vi "Initialize.vi"(4 "stop bits (1.0)":u16(ring)=10 items=["1.0"=10, "2.0"=20], 5 "timeout, ms (300)":u32=300, 6 "parity (none)":enum16{"None", "Odd", "Even"}(ring), 7 "address (1)":u8=1, 8 "error in (no error)":errorcluster, 9 "data bits (8)":u16(ring)=8 items=["7"=7, "8"=8], 10 "baud rate (1200)":u32(ring)=1200 items=["600"=600, "1200"=1200, "2400"=2400, "4800"=4800, "9600"=9600, "19200"=19200], 11 "port":refnum<visa-resource-name>) -> (0 "error out":errorcluster, 3 "HECR out":refnum<class "PL SMC HECR.lvclass">)   [LabVIEW 2015, in "PL SMC HECR.lvclass"]
doc: "Initializes connection to device using specified settings."
uses:
  PL SMC HECR.lvclass
  <vilib>/plasmapper/PL Modbus Client/PL Modbus Client.lvclass
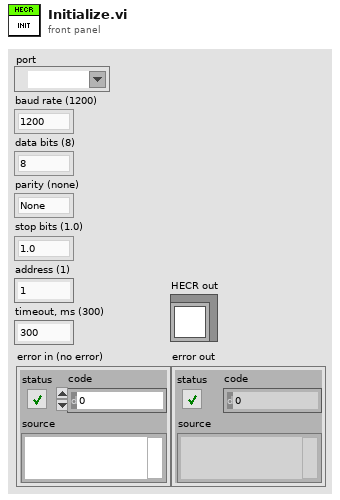
[diagram p1: front panel]
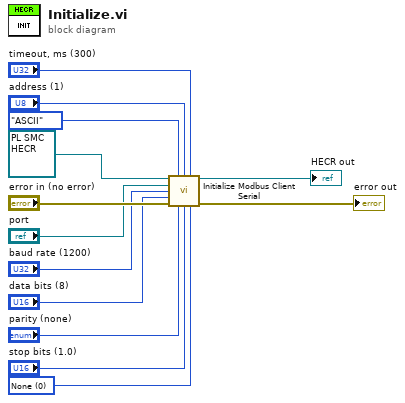
[diagram p0: block diagram]
diagram:
  w9 = u16 0 items=["None", "XON/XOFF", "RTS/CTS", "XON/XOFF & RTS/CTS", "DTR/DSR", "XON/XOFF & DTR/DSR"] ("flow control (none)")
  n1 = call <vilib>:"Initialize Modbus Client Serial.vi"("MODBUS in"=refnum<class "PL SMC HECR.lvclass"> refnum ("Eltochpribor RRG.lvclass"), "protocol (RTU)"=enum16{"RTU", "ASCII", "TCP"}."ASCII", "station address (1)"="address (1)", "timeout, ms (300)"="timeout, ms (300)", "port"="port", "baud rate (9600)"="baud rate (1200)", "data bits (8)"="data bits (8)", "error in (no error)"="error in (no error)", "parity (even)"="parity (none)", "stop bits (1.0)"="stop bits (1.0)", "flow control (none)"=w9) -> ("MODBUS out"=→"HECR out":refnum<class "PL SMC HECR.lvclass">, "error out"=→"error out":errorcluster)  [unwired: 3 in]
